vi "measurement_chart.vi"(8 "error in":errorcluster, 9 "Array of ROI":dbl[][](array[numeric]), 10 "Measurement Chart Settings":T1, 11 "Measurement Chart":refnum<vi>) -> (0 "error out":errorcluster)   [LabVIEW 2012]
uses:
  measurement_graph.ctl
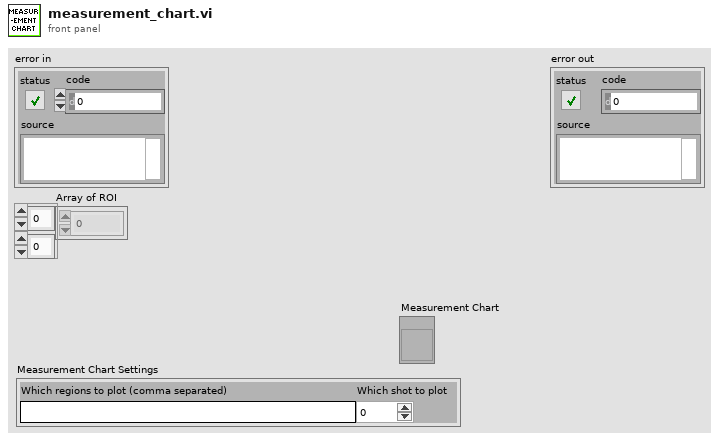
[diagram p1: front panel]
types:
  T1 = typedef "measurement_graph.ctl" = cluster{"Which regions to plot (comma separated)":string, "Which shot to plot":u8}
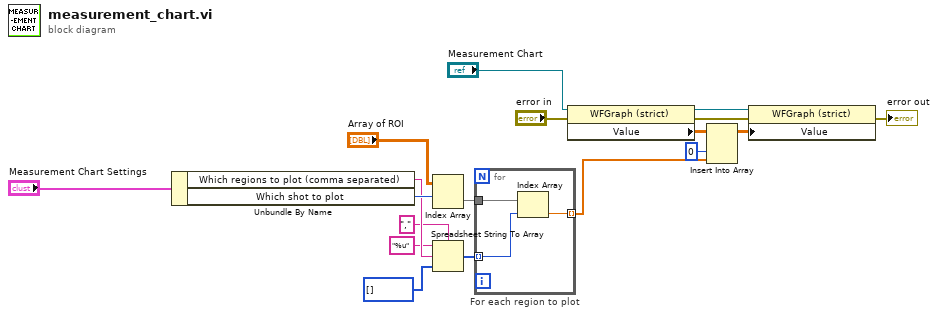
[diagram p0: block diagram]
diagram:
  n1 = Unbundle By Name("Measurement Chart Settings") -> ("Which regions to plot (comma separated)"=w15:string, "Which shot to plot"=w17:u8)
  n2 = Index Array(array="Array of ROI", index (row)=w17) -> (element=w10:dbl[])  [unwired: 1 in]
  n3 = Spreadsheet String To Array(delimiter (Tab)=",", format string="%u", spreadsheet string=w15, array type (2D Dbl)=i32[] []) -> (array=w11:i32[])
  n4 = for "For each region to plot" {
    tunnel: w11 -> [w21] mode=indexing
    tunnel: w10 -> [w20]
    tunnel: [w19] -> w2 mode=indexing
    n5 = Index Array(array=w20, index=w21) -> (element=w19:dbl)
  }
  n6 = property class="WFGraph (strict)"(reference="Measurement Chart", error in="error in") -> (reference out=w3:refnum<vi>, error out=w4:errorcluster, "Value"=w6:dbl[][])
  n7 = Insert Into Array(array=w6, index (col)=0 ("disabled index (col)"), new element=w2) -> (w8:dbl[][])  [unwired: 1 in]
  n8 = property class="WFGraph (strict)"(reference=w3, error in=w4, "Value"=w8) -> (error out=→"error out":errorcluster)  [unwired: 1 out]
